vi "Errorbar0005.vi"   [LabVIEW 2013]
uses:
  <vilib>/Heliosphere Research LLC/Advanced Plotting Toolkit/api_plotting/ErrorbarProperties.ctl
  <vilib>/Heliosphere Research LLC/Advanced Plotting Toolkit/typedefs/PlotColor.ctl
  <vilib>/Heliosphere Research LLC/Advanced Plotting Toolkit/properties/Display.ctl
  ModeType.ctl
  <vilib>/Heliosphere Research LLC/Advanced Plotting Toolkit/api_core/NewPlotScales.ctl
  <vilib>/Heliosphere Research LLC/Advanced Plotting Toolkit/Advanced Plotting Toolkit.lvlib
types:
  T1 = typedef "Advanced Plotting Toolkit.lvlib/NewPlotScales.ctl" = enum16{"Default", "Linear", "Log", "Symlog"}
  T2 = typedef "ModeType.ctl" = enum16{"Normal", "Expected Failure", "Skipped", "Broken"}
  T3 = typedef "Advanced Plotting Toolkit.lvlib/ErrorbarProperties.ctl" = cluster{"Color":T4, "Line Width":dbl, "Cap Size":dbl, "Display":T5}
  T4 = typedef "Advanced Plotting Toolkit.lvlib/PlotColor.ctl" = u32
  T5 = typedef "Advanced Plotting Toolkit.lvlib/Display.ctl" = cluster{"Alpha":dbl, "Z Order":dbl}
  T6 = typedef "Advanced Plotting Toolkit.lvlib/PlotID.ctl" = i32
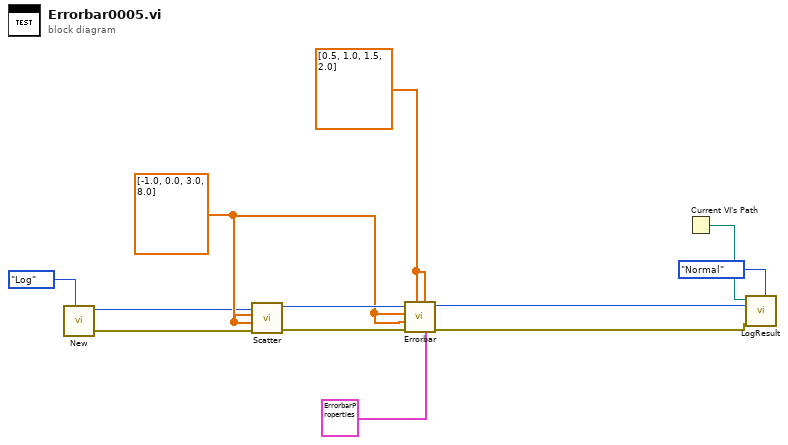
[diagram p0: block diagram]
diagram:
  w6 = dbl[] [0.5, 1.0, 1.5, 2.0] ("X Errors")
  w7 = dbl[] [-1.0, 0.0, 3.0, 8.0] ("X Data")
  n1 = call <vilib>:"New.vi"("X Axis Scale"=NewPlotScales."Log") -> ("error out"=w1:errorcluster, "Plot ID"=w2:T6)  [unwired: 9 in]
  n2 = call <vilib>:"Scatter.vi"("error in (no error)"=w1, "Y Data"=w7, "X Data"=w7, "Plot ID"=w2) -> ("error out"=w8:errorcluster, "Plot ID Out"=w9:T6)  [unwired: 6 in]
  n3 = call <vilib>:"Errorbar.vi"("Properties"=T3 {"Color"=2147483647, "Line Width"=nan, "Cap Size"=nan, "Display"={"Alpha"=nan, "Z Order"=nan}} ("Errorbar Properties"), "Y Errors"=w6, "X Errors"=w6, "error in (no error)"=w8, "Y Data"=w7, "X Data"=w7, "Plot ID"=w9) -> ("error out"=w10:errorcluster, "Plot ID out"=w11:T6)  [unwired: 3 in]
  n4 = Current VI's Path() -> (path=w12:path)
  n5 = call "LogResult.vi"("Mode"=ModeType."Normal", "Test Result"=w10, "Test Artifact"=w11, "VI Path"=w12) -> ()  [unwired: 8 in]
